vi "Send Write Deadband.vi"(7 "Message Priority (Normal)":T2=enum."Normal", 8 "error in (no error)":errorcluster, 10 "Deadband":T1, 11 "Message Enqueuer":refnum<class "Message Enqueuer.lvclass">) -> (0 "error out":errorcluster)   [LabVIEW 2018, in "Level Controller.lvlib" / "Write Deadband Msg.lvclass"]
doc: "This VI sends the message to an actor. The input is the new deadband range. For more information about \"deadband\", see documentation on the Level Controller class."
uses:
  Write Deadband Msg.lvclass
  <vilib>/ActorFramework/Message Enqueuer/Message Enqueuer.lvclass
  <vilib>/ActorFramework/Message Enqueuer/Message Priority.ctl
  Level Controller/Deadband.ctl
  e:/builds/penguin/labview/branches/2018/dev/dist/vi.lib/ActorFramework/Message/Message.lvclass
  Write Deadband Msg.lvclass/Write Deadband Msg.ctl
  <vilib>/ActorFramework/Message Enqueuer/Message Enqueuer.lvclass/Message Enqueuer.ctl
  <vilib>/ActorFramework/Message Priority Queue/Priority Enqueue.vi
  Level Controller/Level Controller.lvclass
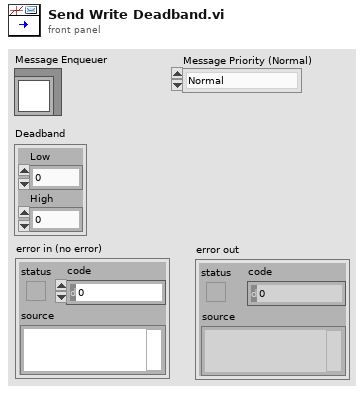
[diagram p1: front panel]
types:
  T1 = typedef "Level Controller.lvlib/Level Controller.lvclass/Deadband.ctl" = cluster{"Low":dbl, "High":dbl}
  T2 = typedef "Actor Framework.lvlib/Message Enqueuer.lvclass/Message Priority.ctl" = enum16{"Low", "Normal", "High"}
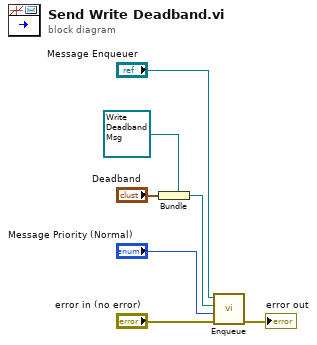
[diagram p0: block diagram]
diagram:
  n1 = Bundle(cluster=refnum<class "Write Deadband Msg.lvclass"> refnum ("Object"), "Deadband") -> (w3:refnum<class "Write Deadband Msg.lvclass">)
  n2 = call <vilib>:"Enqueue.vi"("error in (no error)"="error in (no error)", "Message Priority (Normal)"="Message Priority (Normal)", "Message"=w3, "Message Enqueuer in"="Message Enqueuer") -> ("error out"=→"error out":errorcluster)  [unwired: 6 in, 1 out]
